vi "RobotLiftTeleopCommand.vi"(10 "Buttons":bool[](array[boolean]), 11 "Axes":dbl[](array[numeric])) -> ()   [LabVIEW 2017, in "RobotLift.lvclass"]
uses:
  Subsystem/RobotLift/RobotLift.lvclass
  RobotLiftCommand.ctl
  SubsystemData/RobotLiftData/RobotLiftData.lvclass
  R:/Documents/github/FRC4080/2018-robot-main/SubsystemData/SubsystemData.lvclass
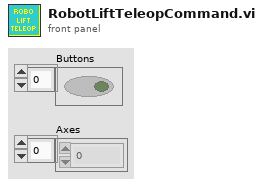
[diagram p1: front panel]
types:
  T1 = typedef "RobotLiftData.lvclass/RobotLiftCommand.ctl" = cluster{"Left Lift":cluster{"Up":bool, "Down":bool}, "Right Lift":cluster{"Up":bool, "Down":bool}, "Release Ramps":bool}
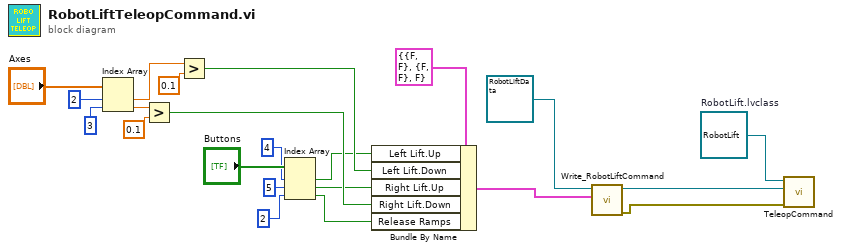
[diagram p0: block diagram]
diagram:
  w4 = refnum<class "RobotLift.lvclass"> refnum  # RobotLift.lvclass
  n1 = Index Array "Index Array"(array="Axes", index #1=2 ("index"), index #2=3 ("index")) -> (element #1=w18:dbl, element #2=w15:dbl)
  n2 = Greater?(x=w15, y=0.1) -> (0:w21:bool)
  n3 = Greater?(x=w18, y=0.1) -> (0:w20:bool)
  n4 = Index Array(array="Buttons", index #1=4 ("index"), index #2=5 ("index"), index #3=2 ("index")) -> (element #1=w7:bool, element #2=w8:bool, element #3=w9:bool)
  n5 = Bundle By Name(cluster=T1 {"Left Lift"={"Up"=FALSE, "Down"=FALSE}, "Right Lift"={"Up"=FALSE, "Down"=FALSE}, "Release Ramps"=FALSE} ("Robot Lift Command"), "Left Lift.Up"=w7, "Left Lift.Down"=w20, "Right Lift.Up"=w8, "Right Lift.Down"=w21, "Release Ramps"=w9) -> (w5:T1)
  n6 = call-dynamic "Write_RobotLiftCommand.vi"("Robot Lift Command"=w5, "RobotLiftData in"=refnum<class "RobotLiftData.lvclass"> refnum) -> ("error out"=w1:errorcluster, "RobotLiftData out"=w3:refnum<class "RobotLiftData.lvclass">)  [unwired: 8 in]
  n7 = call-dynamic "TeleopCommand.vi"("error in (no error)"=w1, "SubsystemData.lvclass"=w3, "Subsystem in"=w4) -> ()  [unwired: 7 in, 2 out]
